vi "NextState.vi"(0 "object in":refnum<class "HaltTactic_v2.lvclass">, 2 "Robot in":refnum<class "Robot.lvclass">, 4 "GameRef":refnum<data-value>, 5 "error in (no error)":errorcluster) -> (14 "object out":refnum<class "HaltTactic_v2.lvclass">, 19 "error out":errorcluster)   [LabVIEW 2023, in "HaltTactic_v2.lvclass"]
uses:
  HaltTactic_v2.lvclass
  Robot_class/Robot.lvclass
  Game_class/Game.lvclass
  Tactic_v2_class/Tactic_v2.lvclass
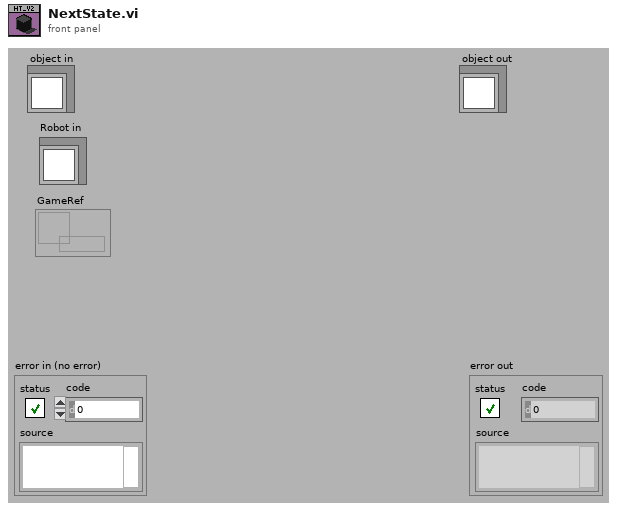
[diagram p1: front panel]
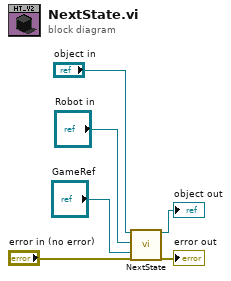
[diagram p0: block diagram]
diagram:
  n1 = call-parent "NextState.vi"("object in"="object in", "Robot in"="Robot in", "GameRef"="GameRef", "error in (no error)"="error in (no error)") -> ("object out"=→"object out":refnum<class "HaltTactic_v2.lvclass">, "error out"=→"error out":errorcluster)  [unwired: 14 in]
